vi "Test Default Audio Device Capture.vi"(8 "error in (no error)":errorcluster) -> (0 "error out":errorcluster, 3 "Pass?":bool)   [LabVIEW 2020]
uses:
  G-Audio/Controls/Backends.ctl
  G-Audio/Controls/Audio Device Info.ctl
  G-Audio/Controls/Audio Device Type.ctl
  8ac02ed0-e0ad-414e-8015-75faf73f9d75.vi
  G-Audio/Private/Result To Error.vi
  8ac02ed0-e0ad-414e-8015-75faf73f9d75.vi/6b901882-6109-4f44-aca5-48e1525e5248.vi
  8ac02ed0-e0ad-414e-8015-75faf73f9d75.vi/06c0137a-63d3-4e30-982f-115d83a1188c.vi
  G-Audio/Private/Get Configured Audio Device Info.vi
  8ac02ed0-e0ad-414e-8015-75faf73f9d75.vi/6b901882-6109-4f44-aca5-48e1525e5248.vi/a9d2058a-38f9-4c88-a1a9-9bf864ebbde5.vi
  8ac02ed0-e0ad-414e-8015-75faf73f9d75.vi/06c0137a-63d3-4e30-982f-115d83a1188c.vi/4b7b629c-2e91-4160-9820-a26af8f6e677.vi
  8ac02ed0-e0ad-414e-8015-75faf73f9d75.vi/06c0137a-63d3-4e30-982f-115d83a1188c.vi/e7c4a249-ce38-42b4-8985-5fdb76b4ebfc.vi
  <vilib>/Utility/Data Type/Get Numeric Information.vi
  <vilib>/Utility/error.llb/Error Cluster From Error Code.vi
  G-Audio/G-Audio.lvlib
panel:
  out "Waveform Graph":waveform(i16)[](graph)
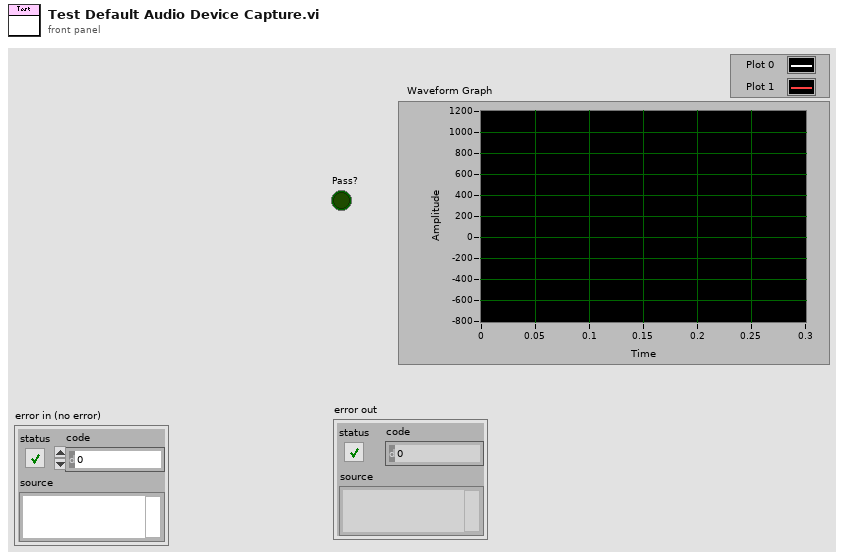
[diagram p1: front panel]
types:
  T1 = typedef "G-Audio.lvlib/Backends.ctl" = enum16{"WASAPI", "DirectSound", "WinMM", "Core Audio", "sndio", "audio(4)", "OSS", "PulseAudio", "ALSA", "JACK", "AAudio", "OpenSL|ES", "Web Audio", "Custom", "Null", "Default"}
  T2 = typedef "G-Audio.lvlib/Audio Device Info.ctl" = cluster{"Name":string, "ID":u8[], "Device Type":T3}
  T3 = typedef "G-Audio.lvlib/Audio Device Type.ctl" = enum16{"(None)", "Playback", "Capture", "Duplex", "Loopback"}
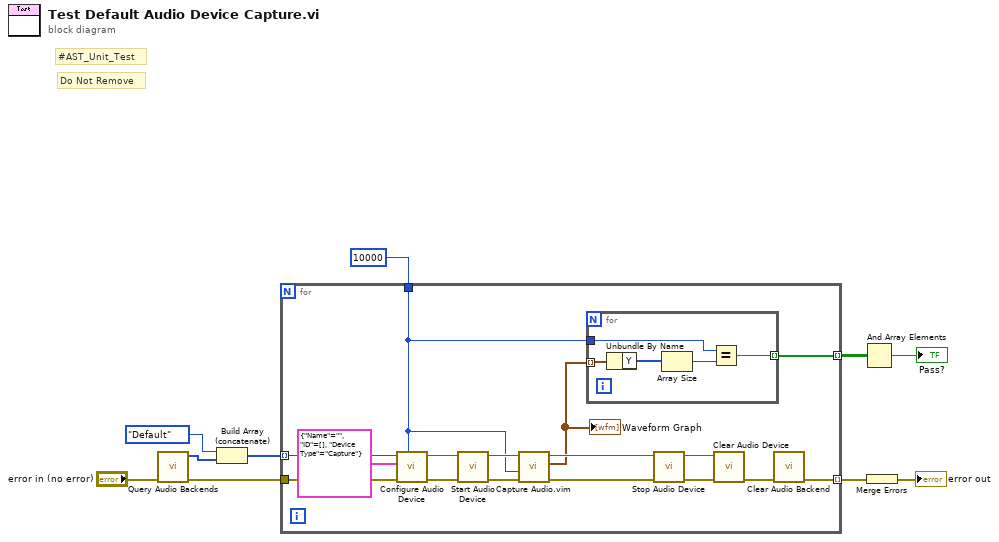
[diagram p0: block diagram]
diagram:
  # "Do Not Remove"
  # "#AST_Unit_Test"
  n1 = call "Query Audio Backends.vi"("error in (no error)"="error in (no error)") -> ("error out"=w9:errorcluster, "Backends"=w8:T1[])  [unwired: 9 in]
  n2 = Build Array (concatenate)(Backends."Default" ("Backends"), w8) -> (w6:T1[])
  n3 = for {
    tunnel: w9 -> [w19]
    tunnel: w6 -> [w18] mode=indexing
    tunnel: [w14] -> w5 mode=indexing
    tunnel: 10000 -> [w12]
    tunnel: [w11] -> w2 mode=indexing
    n4 = call "Configure Audio Device.vi"("Buffer Size (4096)"=w12, "error in (no error)"=w19, "Audio Device"=T2 {"Name"="", "ID"=[], "Device Type"=enum."Capture"}, "Backend (Default)"=w18) -> ("error out"=w25:errorcluster, "Audio Device Refnum"=w26:refnum<file>)  [unwired: 6 in]
    n5 = call "Start Audio Device.vi"("error in (no error)"=w25, "Audio Device Refnum In"=w26) -> ("error out"=w23:errorcluster, "Audio Device Refnum Out"=w24:refnum<file>)  [unwired: 8 in]
    n6 = call "Capture Audio.vim"("error in (no error)"=w23, "Samples To Read"=w12, "Audio Device Refnum In"=w24) -> ("error out"=w15:errorcluster, "Audio Data"=w13:waveform(i16)[], "Audio Device Refnum Out"=w16:refnum<file>)  [unwired: 6 in]
    "Waveform Graph" <- w13
    n7 = for {
      tunnel: w13 -> [w31] mode=indexing
      tunnel: w12 -> [w29]
      tunnel: [w27] -> w11 mode=indexing
      n8 = Unbundle By Name(w31) -> ("Y"=w30:i16[])
      n9 = Array Size(array=w30) -> (size(s)=w28:i32)
      n10 = Equal?(x=w29, y=w28) -> (x = y?=w27:bool)
    }
    n11 = call "Stop Audio Device.vi"("error in (no error)"=w15, "Audio Device Refnum In"=w16) -> ("error out"=w21:errorcluster, "Audio Device Refnum Out"=w20:refnum<file>)  [unwired: 8 in]
    n12 = call "Clear Audio Device.vi"("error in (no error)"=w21, "Audio Device Refnum In"=w20) -> ("error out"=w22:errorcluster)  [unwired: 9 in]
    n13 = call "Clear Audio Backend.vi"("error in (no error)"=w22) -> ("error out"=w14:errorcluster)  [unwired: 10 in]
  }
  n14 = And Array Elements(Boolean array=w2) -> (logical AND=→"Pass?":bool)
  n15 = Merge Errors(w5) -> (→"error out":errorcluster)
